vi "DG645_control.vi"() -> ()   [LabVIEW 2015]
uses:
  <vilib>/Utility/xml.llb/Write to XML File(string).vi
  <vilib>/Utility/xml.llb/Read From XML File(string).vi
  <instrlib>/Stanford Research DG645/Stanford Research DG645.lvlib
panel:
  out "Digital Waveform Graph":digitalwaveform(graph)={"t0"=timestamp(0 s since 1904-01-01), "dt"=4.817138671875e-08, "Y"={"transitions"=[], "data"=array4096x5[20480 elements]}}
  out "Updating":bool
  out "Error":bool
  in  "Reset on update?":bool
  in  "Stop":bool
  in  "Trigger Source":u16(ring)=6 items=["Internal", "External rising edge", "External falling edge", "Single shot internal rising edge", "Single shot external rising edge", "Single shot", "Line"]
  in  "Export to File":bool
  in  "Import From File":bool
  in  "Update Device":bool
  out "error out":errorcluster
  in  "Delays":T1(array[cluster])=[{"Channel"=2, "Reference"=0, "Delay Time"=1e-08}, {"Channel"=3, "Reference"=2, "Delay Time"=1e-05}, {"Channel"=4, "Reference"=2, "Delay Time"=0.000186}, {"Channel"=5, "Reference"=4, "Delay Time"=1e-05}, {"Channel"=6, "Reference"=4, "Delay Time"=3e-07}, {"Channel"=7, "Reference"=6, "Delay Time"=1e-05}, {"Channel"=8, "Reference"=6, "Delay Time"=1e-06}, {"Channel"=9, "Reference"=8, "Delay Time"=1e-05}] {"Delay Time" format="%#_6p"; "Reference" items=["T0"=0, "A"=2, "B"=3, "C"=4, "D"=5, "E"=6, "F"=7, "G"=8, "H"=9]; "Channel" items=["A"=2, "B"=3, "C"=4, "D"=5, "E"=6, "F"=7, "G"=8, "H"=9]}
  in  "Trigger Rate":dbl=50.0
  in  "Outputs":T2(array[cluster])=[{"Output"=0, "Offset"=0.0, "Level"=5.0, "Polarity"=TRUE, "Prescale Factor"=2, "Prescale Phase"=0, "Description"="valve"}, {"Output"=1, "Offset"=0.0, "Level"=5.0, "Polarity"=TRUE, "Prescale Factor"=1, "Prescale Phase"=0, "Description"="flash lamp"}, {"Output"=2, "Offset"=0.0, "Level"=2.7, "Polarity"=TRUE, "Prescale Factor"=1, "Prescale Phase"=0, "Description"="q-switch"}, {"Output"=3, "Offset"=0.0, "Level"=5.0, "Polarity"=TRUE, "Prescale Factor"=1, "Prescale Phase"=0, "Description"="ramp"}, {"Output"=4, "Offset"=0.0, "Level"=5.0, "Polarity"=TRUE, "Prescale Factor"=1, "Prescale Phase"=0, "Description"="scope"}] {"Output" items=["T0", "Output AB", "Output CD", "Output EF", "Output GH"]; "Offset" format="%#_13g"; "Prescale Phase" max=1073741822; "Prescale Factor" min=1 max=1073741823}
  in  "VISA resource name":refnum<visa-resource-name>="DG645_HOGAN"
  # "DG645 control"
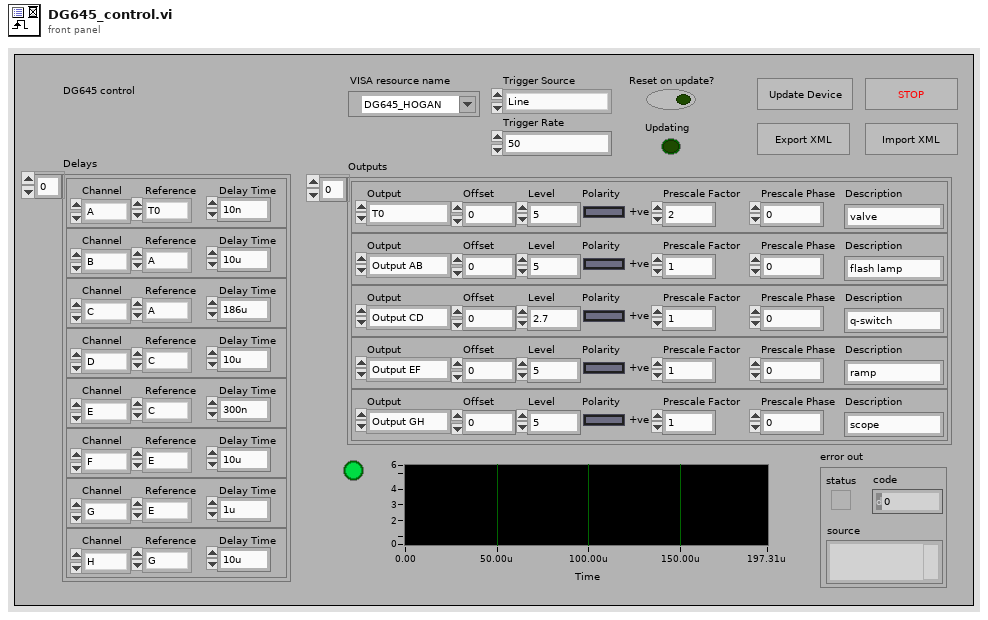
[diagram p1: front panel]
types:
  T1 = cluster{"Channel":u16, "Reference":u16, "Delay Time":dbl}[]
  T2 = cluster{"Output":u16, "Offset":dbl, "Level":dbl, "Polarity":bool, "Prescale Factor":u32, "Prescale Phase":u32, "Description":string}[]
  T3 = cluster{"VISA resource name":refnum<visa-resource-name>, "Trigger Source":u16, "Trigger Rate":dbl, "Delays":cluster{"Channel":u16, "Reference":u16, "Delay Time":dbl}[], "Outputs":cluster{"Output":u16, "Offset":dbl, "Level":dbl, "Polarity":bool, "Prescale Factor":u32, "Prescale Phase":u32, "Description":string}[]}
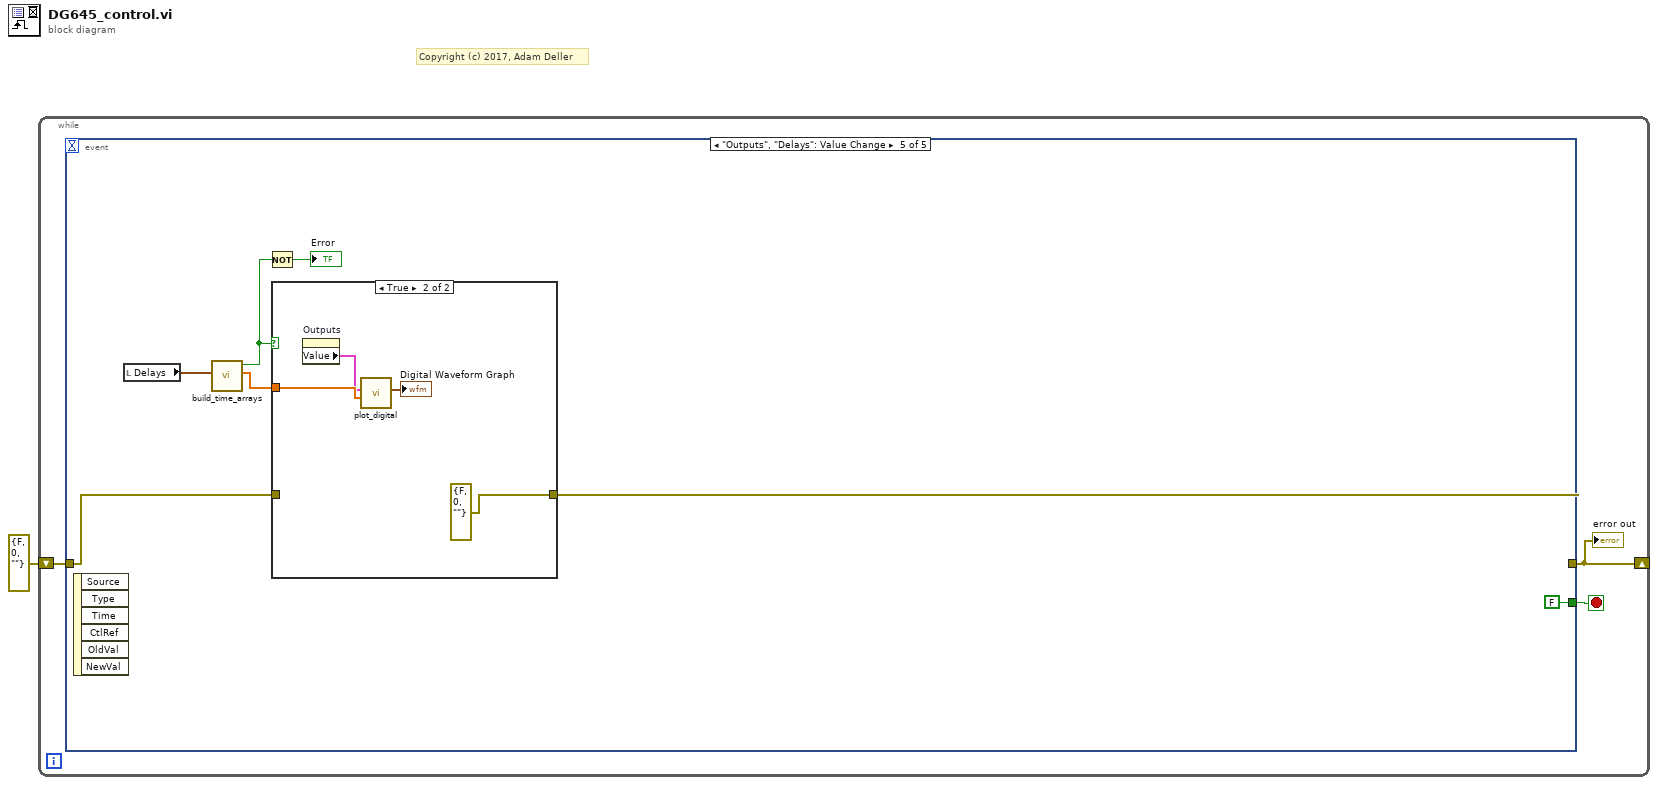
[diagram p0: block diagram]
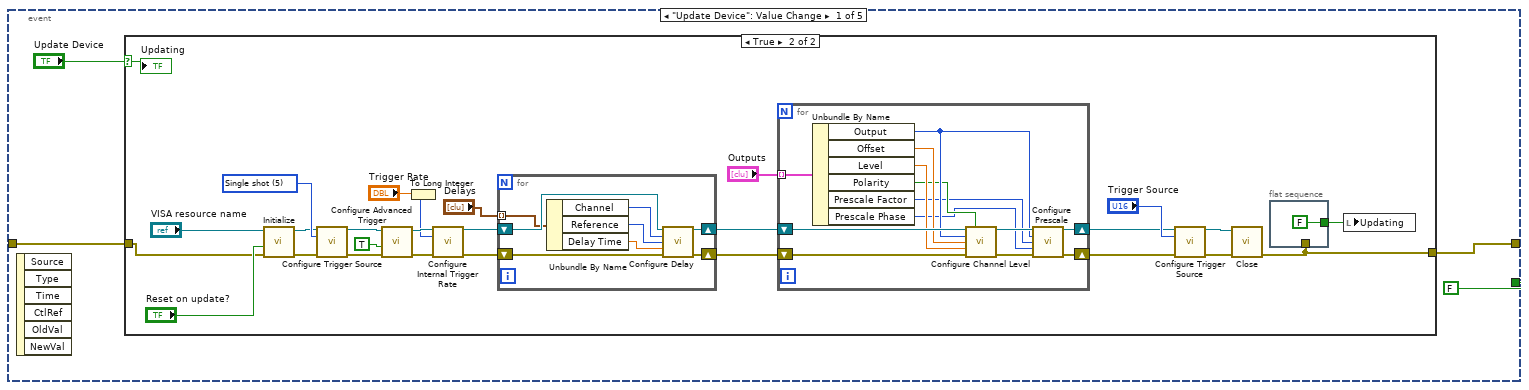
[diagram p2: hidden frame]
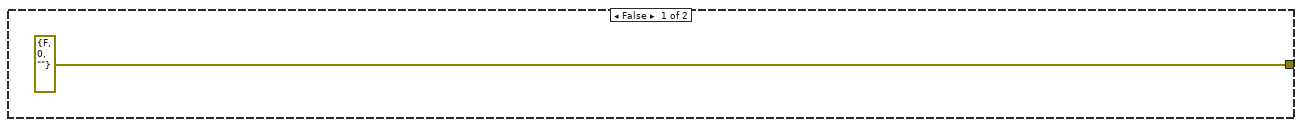
[diagram p3: hidden frame]
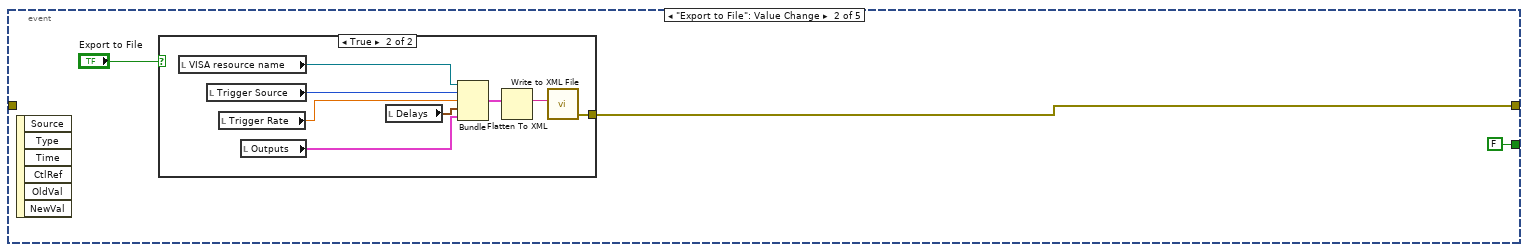
[diagram p4: hidden frame]
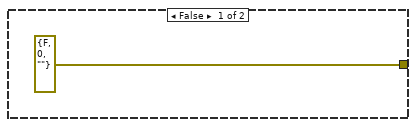
[diagram p5: hidden frame]
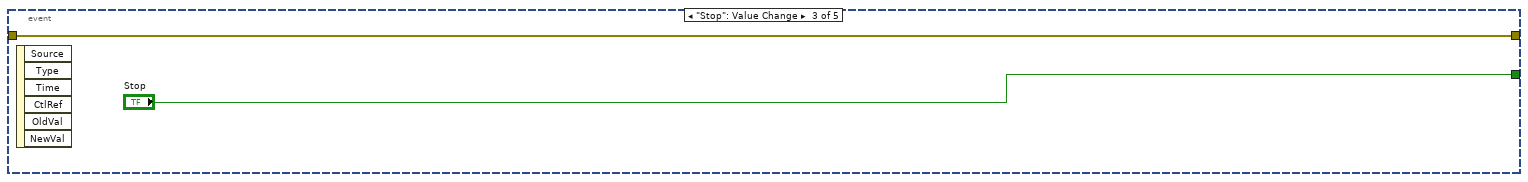
[diagram p6: hidden frame]
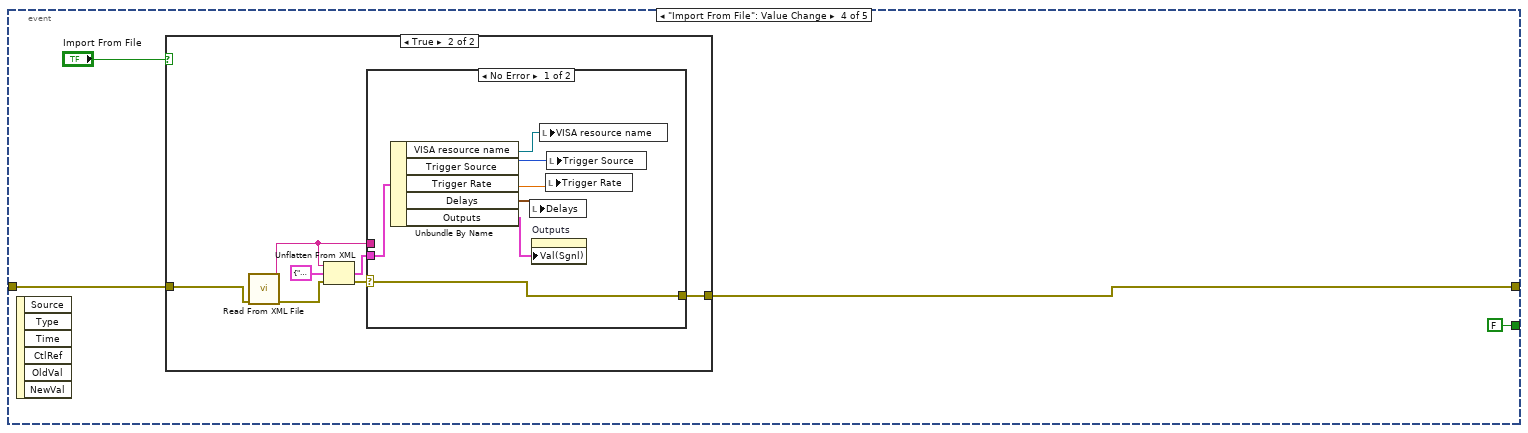
[diagram p7: hidden frame]
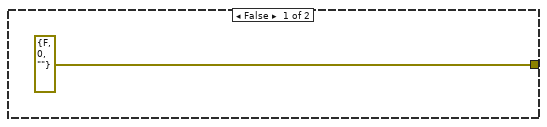
[diagram p8: hidden frame]
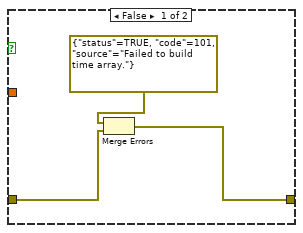
[diagram p10: hidden frame]
diagram:
  # "Copyright (c) 2017, Adam Deller"
  n1 = while {
    shift-right: [w3] -> _
    shift-left: errorcluster {"status"=FALSE, "code"=0, "source"=""} ("error out") -> [w2]
    stop <- w4 stop-if-true
    n2 = event shown="[4] \"Outputs\", \"Delays\": Value Change" {
      selector: _ -> [_ _ _ _ _]
      dyn-events: _ -> [_ _ _ _ _]
      timeout: _ -> [_ _ _ _ _]
      tunnel: [w8 w61 w71 w76 w98] -> w3
      tunnel: [FALSE ("Stop") FALSE ("Stop") "Stop" FALSE ("Stop") FALSE ("Stop")] -> w4
      tunnel: w2 -> [w5 _ w71 w73 w93]
      event "Update Device": Value Change {
        n3 = event-data() -> ()  [unwired: 1 in, 6 out]
        n4 = case shown="True" "Update Device" {
          selector: "Update Device" -> [_ w15]
          tunnel: [errorcluster {"status"=FALSE, "code"=0, "source"=""} ("error out") w14] -> w8
          tunnel: w5 -> [_ w10]
          frame False {
          }
          frame True {
            w23 = u16 5 items=["Internal", "External rising edge", "External falling edge", "Single shot internal rising edge", "Single shot external rising edge", "Single shot", "Line"] ("Trigger Source (5:Single Shot)")
            n5 = call <instrlib>:"Initialize.vi"("error in (no error)"=w10, "Reset (True)"="Reset on update?", "VISA resource name"="VISA resource name") -> ("error out"=w22:errorcluster, "VISA resource name out"=w21:refnum<visa-resource-name>)  [unwired: 7 in]
            n6 = call <instrlib>:"Configure Trigger Source.vi"("VISA resource name"=w21, "Trigger Source (5:Single Shot)"=w23, "error in (no error)"=w22) -> ("VISA resource name out"=w20:refnum<visa-resource-name>, "error out"=w19:errorcluster)  [unwired: 11 in]
            n7 = call <instrlib>:"Configure Advanced Trigger.vi"("error in (no error)"=w19, "Enable Advanced Trigger (False)"=TRUE, "VISA resource name"=w20) -> ("error out"=w29:errorcluster, "VISA resource name out"=w28:refnum<visa-resource-name>)  [unwired: 7 in]
            n8 = To Long Integer(number="Trigger Rate") -> (32bit integer=w11:i32)
            n9 = call <instrlib>:"Configure Internal Trigger Rate.vi"("VISA resource name"=w28, "Internal Trigger Rate (1 MHz)"=w11, "error in (no error)"=w29) -> ("VISA resource name out"=w30:refnum<visa-resource-name>, "error out"=w32:errorcluster)  [unwired: 11 in]
            n10 = for {
              tunnel: "Delays" -> [w43] mode=indexing
              shift-right: [w39] -> w18
              shift-left: w30 -> [w45]
              shift-right: [w38] -> w17
              shift-left: w32 -> [w44]
              n11 = Unbundle By Name(w43) -> ("Channel"=w42:u16, "Reference"=w41:u16, "Delay Time"=w40:dbl)
              n12 = call <instrlib>:"Configure Delay.vi"("VISA resource name"=w45, "Channel to Modify (2:A)"=w42, "Reference Channel (0:T0)"=w41, "Delay Time (0 s)"=w40, "error in (no error)"=w44) -> ("VISA resource name out"=w39:refnum<visa-resource-name>, "error out"=w38:errorcluster)  [unwired: 9 in]
            }
            n13 = for {
              shift-right: [w56] -> w26
              shift-left: w17 -> [w58]
              tunnel: "Outputs" -> [w55] mode=indexing
              shift-right: [w46] -> w16
              shift-left: w18 -> [w57]
              n14 = Unbundle By Name(w55) -> ("Output"=w53:u16, "Offset"=w52:dbl, "Level"=w51:dbl, "Polarity"=w50:bool, "Prescale Factor"=w49:u32, "Prescale Phase"=w48:u32)
              n15 = call <instrlib>:"Configure Channel Level.vi"("VISA resource name"=w57, "Positive Level Polarity (True)"=w50, "Output Channel (0:T0)"=w53, "Level Offset (0 V)"=w52, "Level Amplitude (2.5 V)"=w51, "error in (no error)"=w58) -> ("VISA resource name out"=w54:refnum<visa-resource-name>, "error out"=w47:errorcluster)  [unwired: 8 in]
              n16 = call <instrlib>:"Configure Prescale.vi"("VISA resource name"=w54, "Output Channel (0:T0)"=w53, "Prescale Factor (1)"=w49, "Prescale Phase (0)"=w48, "error in (no error)"=w47) -> ("VISA resource name out"=w46:refnum<visa-resource-name>, "error out"=w56:errorcluster)  [unwired: 9 in]
            }
            n17 = call <instrlib>:"Configure Trigger Source.vi"("VISA resource name"=w16, "Trigger Source (5:Single Shot)"="Trigger Source", "error in (no error)"=w26) -> ("VISA resource name out"=w25:refnum<visa-resource-name>, "error out"=w27:errorcluster)  [unwired: 11 in]
            n18 = call <instrlib>:"Close.vi"("error in (no error)"=w27, "VISA resource name"=w25) -> ("error out"=w14:errorcluster)  [unwired: 9 in]
            n19 = flat-sequence {
              tunnel: w14 -> [_]
              tunnel: [FALSE ("Boolean")] -> w13
              frame #0 {
              }
            }
            n20 = local write "Updating"(w13) -> ()
            "Updating" <- w15
          }
        }
      }
      event "Export to File": Value Change {
        n21 = event-data() -> ()  [unwired: 1 in, 6 out]
        n22 = case shown="True" "Export to File" {
          tunnel: [errorcluster {"status"=FALSE, "code"=0, "source"=""} ("error out") w63] -> w61
          frame False {
          }
          frame True {
            n23 = local read "VISA resource name"() -> (w70:refnum<visa-resource-name>)
            n24 = local read "Trigger Source"() -> (w69:u16)
            n25 = local read "Trigger Rate"() -> (w68:dbl)
            n26 = local read "Outputs"() -> (w66:T2)
            n27 = local read "Delays"() -> (w67:T1)
            n28 = Bundle("VISA resource name"=w70, "Trigger Source"=w69, "Trigger Rate"=w68, "Delays"=w67, "Outputs"=w66) -> (w65:T3)  [unwired: 1 in]
            n29 = Flatten To XML(anything=w65) -> (xml string=w64:string)
            n30 = call-poly <vilib>:"Write to XML File.vi"("XML Input"=w64) -> ("error out"=w63:errorcluster)  [unwired: 8 in, 2 out]
          }
        }
      }
      event "Stop": Value Change {
        n31 = event-data() -> ()  [unwired: 1 in, 6 out]
      }
      event "Import From File": Value Change {
        n32 = event-data() -> ()  [unwired: 1 in, 6 out]
        n33 = case shown="True" "Import From File" {
          tunnel: [errorcluster {"status"=FALSE, "code"=0, "source"=""} ("error out") w81] -> w76
          tunnel: w73 -> [_ w78]
          frame False {
          }
          frame True {
            n34 = call-poly <vilib>:"Read From XML File.vi"("error in (no error)"=w78) -> ("error out"=w80:errorcluster, "XML Elements"=w79:string)  [unwired: 8 in, 1 out]
            n35 = Unflatten From XML(xml string=w79, type=T3 {"VISA resource name"="", "Trigger Source"=0, "Trigger Rate"=0.0, "Delays"=[], "Outputs"=[]} ("output cluster"), error in (no error)=w80) -> (value=w83:T3, error out=w82:errorcluster)
            n36 = case shown="No Error" w82 {
              selector: w82 -> [w90 w92]
              tunnel: w83 -> [w91 _]
              tunnel: [w90 w92] -> w81
              tunnel: w79 -> [_ _]
              frame No Error {
                n37 = Unbundle By Name(w91) -> ("VISA resource name"=w89:refnum<visa-resource-name>, "Trigger Source"=w88:u16, "Trigger Rate"=w87:dbl, "Delays"=w86:T1, "Outputs"=w85:T2)
                n38 = local write "Delays"(w86) -> ()
                n39 = property on="Outputs" class="Arr (strict)"("Val(Sgnl)"=w85) -> ()  [unwired: 2 in, 2 out]
                n40 = local write "VISA resource name"(w89) -> ()
                n41 = local write "Trigger Rate"(w87) -> ()
                n42 = local write "Trigger Source"(w88) -> ()
              }
              frame Error {
              }
            }
          }
        }
      }
      event "Outputs", "Delays": Value Change {
        n43 = event-data() -> ()  [unwired: 1 in, 6 out]
        n44 = local read "Delays"() -> (w97:T1)
        n45 = call "build_time_arrays.vi"("Delays"=w97) -> ("Array"=w96:dbl[], "ok"=w95:bool)  [unwired: 9 in]
        n46 = Not(x=w95) -> (.not. x?=→"Error":bool)
        n47 = case shown="True" w95 {
          tunnel: w96 -> [_ w105]
          tunnel: [w101 errorcluster {"status"=FALSE, "code"=0, "source"=""} ("error out")] -> w98
          tunnel: w93 -> [w102 _]
          frame False {
            n48 = Merge Errors(errorcluster {"status"=TRUE, "code"=101, "source"="Failed to build time array."} ("error out"), w102) -> (w101:errorcluster)
          }
          frame True {
            n49 = property on="Outputs" class="Arr (strict)"() -> ("Value"=w104:T2)  [unwired: 2 in, 2 out]
            n50 = call "plot_digital.vi"("array"=w105, "Outputs"=w104) -> ("Digital Waveform Graph"=→"Digital Waveform Graph":digitalwaveform)  [unwired: 9 in]
          }
        }
      }
    }
    "error out" <- w3
  }
